vi "Configure Pulse.vi"(0 "VISA resource name":refnum<visa-resource-name>, 1 "Pulse Width (0)":dbl, 2 "Rising Edge Time (1.9531E-6 s)":dbl=1.9531e-06, 5 "Output Channel (1: Channel 1)":i32(ring)=1 items=["Channel 1"=1, "Channel 2"=2], 7 "Pulse Hold (1: Duty)":i32(ring)=1 items=["Width", "Duty"], 9 "Delay (0 s)":dbl, 11 "error in (no error)":errorcluster, 12 "Duty Cycle (50 %)":dbl=50.0, 13 "Falling Edge Time (1.9531E-6 s)":dbl=1.9531e-06) -> (4 "VISA resource name out":refnum<visa-resource-name>, 15 "error out":errorcluster)   [LabVIEW 2015, in "RIGOL DG4000 Series.lvlib"]
doc: "Configure pulse settings."
uses:
  <instrlib>/RIGOL DG4000 Series/RIGOL DG4000 Series.lvlib
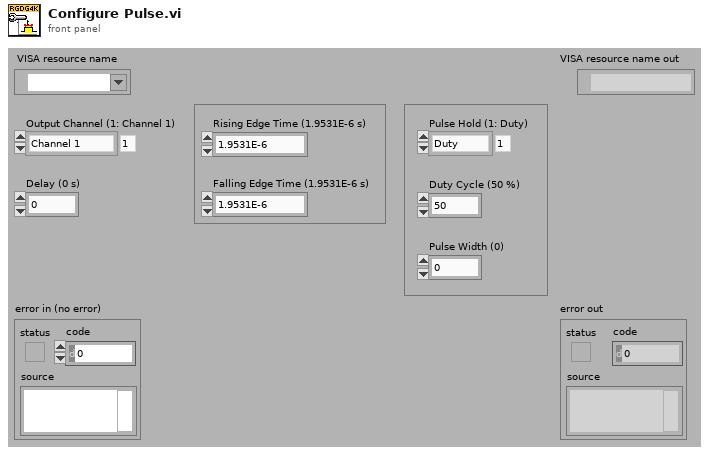
[diagram p1: front panel]
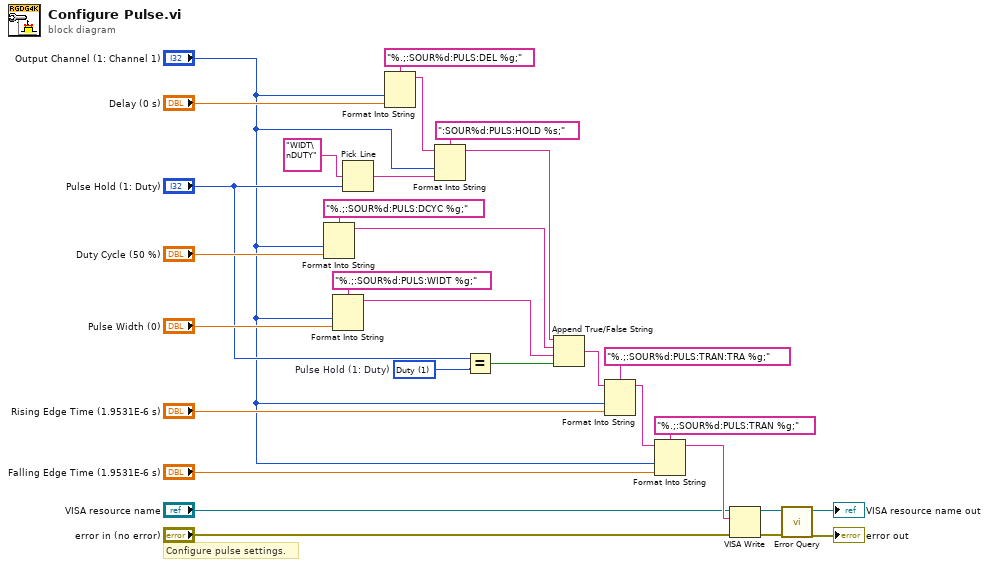
[diagram p0: block diagram]
diagram:
  w3 = 1 items=["Width", "Duty"]  # Pulse Hold (1: Duty)
  # "Configure pulse settings."
  n1 = Format Into String(format string="%.;:SOUR%d:PULS:DCYC %g;", "Output Channel (1: Channel 1)", "Duty Cycle (50 %)") -> (resulting string=w6:string)  [unwired: 2 in, 1 out]
  n2 = Format Into String(format string="%.;:SOUR%d:PULS:WIDT %g;", "Output Channel (1: Channel 1)", "Pulse Width (0)") -> (resulting string=w5:string)  [unwired: 2 in, 1 out]
  n3 = Pick Line(multi-line string="WIDT\nDUTY", line index="Pulse Hold (1: Duty)") -> (output string=w23:string)  [unwired: 1 out]
  n4 = Format Into String(format string="%.;:SOUR%d:PULS:DEL %g;", "Output Channel (1: Channel 1)", "Delay (0 s)") -> (resulting string=w25:string)  [unwired: 2 in, 1 out]
  n5 = Format Into String(format string=":SOUR%d:PULS:HOLD %s;", initial string=w25, "Output Channel (1: Channel 1)", w23) -> (resulting string=w7:string)  [unwired: 1 in, 1 out]
  n6 = Equal?(x="Pulse Hold (1: Duty)", y=w3) -> (x = y?=w4:bool)
  n7 = Append True/False String(1:w4, 2:w5, 3:w6, 4:w7) -> (0:w8:string)
  n8 = Format Into String(format string="%.;:SOUR%d:PULS:TRAN:TRA %g;", initial string=w8, "Output Channel (1: Channel 1)", "Rising Edge Time (1.9531E-6 s)") -> (resulting string=w18:string)  [unwired: 1 in, 1 out]
  n9 = Format Into String(format string="%.;:SOUR%d:PULS:TRAN %g;", initial string=w18, "Output Channel (1: Channel 1)", "Falling Edge Time (1.9531E-6 s)") -> (resulting string=w15:string)  [unwired: 1 in, 1 out]
  n10 = VISA Write(VISA resource name="VISA resource name", write buffer=w15, error in (no error)="error in (no error)") -> (VISA resource name out=w12:refnum<visa-resource-name>, error out=w11:errorcluster)  [unwired: 1 out]
  n11 = call <instrlib>:"Error Query.vi"("error in (no error)"=w11, "VISA resource name"=w12) -> ("error out"=→"error out":errorcluster, "VISA resource name out"=→"VISA resource name out":refnum<visa-resource-name>)  [unwired: 8 out]
